vi "angle_corrector_array.vi"(10 "angle":dbl) -> (2 "angle corrected":dbl)   [LabVIEW 2020]
panel:
  # "Angle corrector"
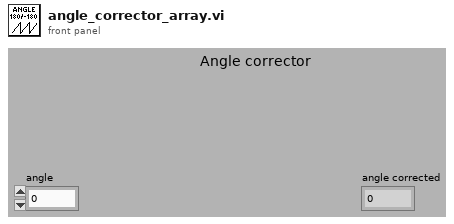
[diagram p1: front panel]
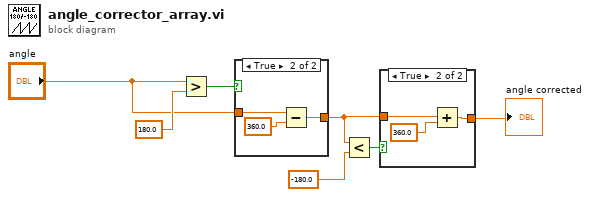
[diagram p0: block diagram]
diagram:
  n1 = Greater?(x="angle", y=180.0) -> (0:w5:bool)
  n2 = case shown="True" w5 {
    tunnel: "angle" -> [w8 w10]
    tunnel: [w8 w9] -> w3
    frame False {
    }
    frame True {
      n3 = Subtract(x=w10, y=360.0) -> (x-y=w9:dbl)
    }
  }
  n4 = Less?(x=w3, y=-180.0) -> (x < y?=w4:bool)
  n5 = case shown="True" w4 {
    tunnel: w3 -> [w12 w14]
    tunnel: [w12 w13] -> w2
    frame False {
    }
    frame True {
      n6 = Add(x=w14, y=360.0) -> (x+y=w13:dbl)
    }
  }
  "angle corrected" <- w2
